vi "1st Derivative of Rational Polynomial (CDB).vi"(9 "GCD?":bool=TRUE, 10 "Q(x)":cdb[](array[numeric]) format="%#.6g", 11 "P(x)":cdb[](array[numeric]) format="%#.6g") -> (0 "error":i32, 2 "Denominator d[P(x)/Q(x)]/dx":cdb[](array[numeric]), 3 "Numerator d[P(x)/Q(x)]/dx":cdb[](array[numeric]))   [LabVIEW 2017, in "NI_AALPro.lvlib"]
uses:
  NI_AALPro.lvlib
  GCD of P(x) and Q(x) (CDB).vi
  Subtract Polynomials (CDB).vi
  Multiply Polynomials (CDB).vi
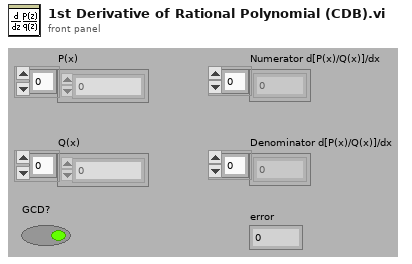
[diagram p1: front panel]
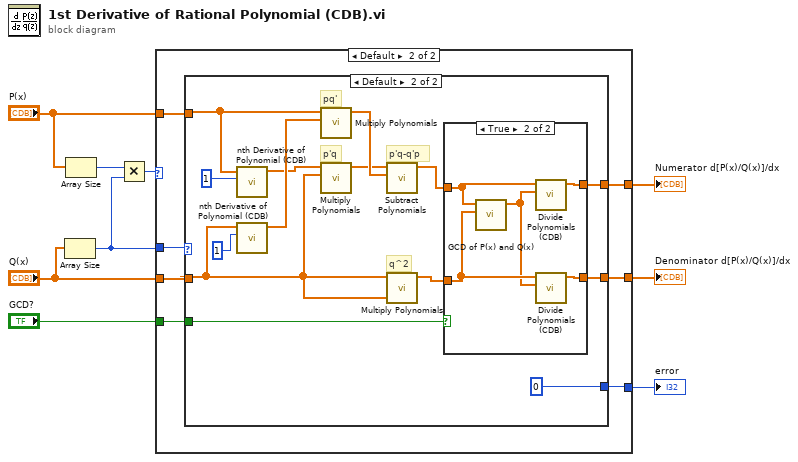
[diagram p0: block diagram]
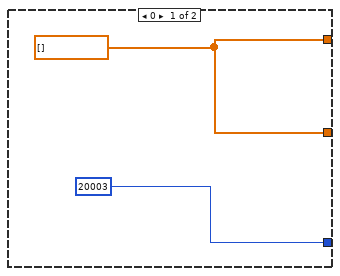
[diagram p2: hidden frame]
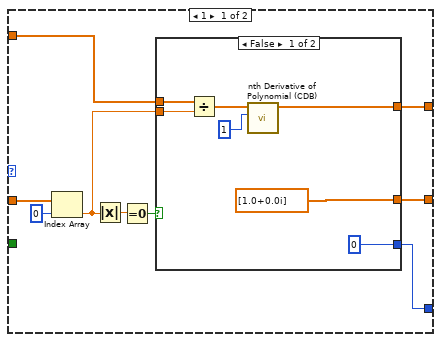
[diagram p3: hidden frame]
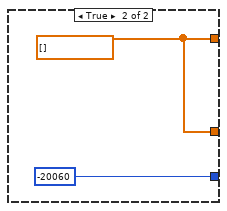
[diagram p4: hidden frame]
diagram:
  n1 = Array Size(array="Q(x)") -> (size(s)=w3:i32)
  n2 = Array Size(array="P(x)") -> (size(s)=w4:i32)
  n3 = Multiply(x=w4, y=w3) -> (x*y=w2:i32)
  n4 = case shown="Default" w2 {
    tunnel: "P(x)" -> [_ w15]
    tunnel: [w11 w17] -> w9
    tunnel: [w11 w16] -> w8
    tunnel: "Q(x)" -> [_ w18]
    tunnel: [20003 ("empty array") w14] -> w6
    tunnel: w3 -> [_ w13]
    tunnel: "GCD?" -> [_ w12]
    frame 0 {
      w11 = cdb[] []
    }
    frame Default {
      n5 = case shown="Default" w13 {
        tunnel: w18 -> [w27 w44]
        tunnel: [w24 w43] -> w17
        tunnel: [w23 w42] -> w16
        tunnel: w15 -> [w22 w45]
        tunnel: [w21 0] -> w14
        tunnel: w12 -> [_ w37]
        frame 1 {
          n6 = Index Array(array=w27, index=0) -> (element=w20:cdb)
          n7 = Absolute Value(x=w20) -> (abs(x)=w19:dbl)
          n8 = Equal To 0?(x=w19) -> (x = 0?=w25:bool)
          n9 = case shown="False" w25 {
            tunnel: [w31 w36] -> w24
            tunnel: [cdb[] [1.0+0.0i] w36] -> w23
            tunnel: w22 -> [w34 _]
            tunnel: w20 -> [w33 _]
            tunnel: [0 ("divide by zero") -20060 ("divide by zero")] -> w21
            frame False {
              n10 = Divide(x=w34, y=w33) -> (x/y=w32:cdb[])
              n11 = call "nth Derivative of Polynomial (CDB).vi"("order"=1, "P(x)"=w32) -> ("Nth Derivative of P(x)"=w31:cdb[])  [unwired: 8 in, 1 out]
            }
            frame True {
              w36 = cdb[] []
            }
          }
        }
        frame Default {
          # "q^2"
          # "p'q"
          # "pq'"
          # "p'q-q'p"
          n12 = call "nth Derivative of Polynomial (CDB).vi"("order"=1, "P(x)"=w45) -> ("Nth Derivative of P(x)"=w49:cdb[])  [unwired: 8 in, 1 out]
          n13 = call "nth Derivative of Polynomial (CDB).vi"("order"=1, "P(x)"=w44) -> ("Nth Derivative of P(x)"=w50:cdb[])  [unwired: 8 in, 1 out]
          n14 = call-poly "Multiply Polynomials.vi"("Q(x)"=w50, "P(x)"=w45) -> ("P(x)*Q(x)"=w48:cdb[])  [unwired: 8 in, 1 out]
          n15 = call-poly "Multiply Polynomials.vi"("Q(x)"=w44, "P(x)"=w49) -> ("P(x)*Q(x)"=w40:cdb[])  [unwired: 8 in, 1 out]
          n16 = call-poly "Subtract Polynomials.vi"("Q(x)"=w48, "P(x)"=w40) -> ("P(x)-Q(x)"=w47:cdb[])  [unwired: 8 in, 1 out]
          n17 = call-poly "Multiply Polynomials.vi"("Q(x)"=w44, "P(x)"=w44) -> ("P(x)*Q(x)"=w46:cdb[])  [unwired: 8 in, 1 out]
          n18 = case shown="True" w37 {
            tunnel: w47 -> [w52 w55]
            tunnel: w46 -> [w51 w54]
            tunnel: [w52 w57] -> w43
            tunnel: [w51 w56] -> w42
            frame False {
            }
            frame True {
              n19 = call-poly "GCD of P(x) and Q(x).vi"("Q(x)"=w54, "P(x)"=w55) -> ("Greatest Common Divisor"=w53:cdb[])  [unwired: 8 in, 1 out]
              n20 = call "Divide Polynomials (CDB).vi"("Q(x)"=w53, "P(x)"=w55) -> ("P(x)/Q(x)"=w57:cdb[])  [unwired: 7 in, 2 out]
              n21 = call "Divide Polynomials (CDB).vi"("Q(x)"=w53, "P(x)"=w54) -> ("P(x)/Q(x)"=w56:cdb[])  [unwired: 7 in, 2 out]
            }
          }
        }
      }
    }
  }
  "Numerator d[P(x)/Q(x)]/dx" <- w9
  "Denominator d[P(x)/Q(x)]/dx" <- w8
  "error" <- w6
